vi "Regulator.vi"(8 "Odczyt odom":bool, 9 "Parametry regulatora":cluster{"kp":dbl, "k alfa":dbl, "k beta":dbl}, 10 "Odległość do punktu":dbl format="%#_13g", 11 "Kąt tryg. zad":dbl) -> (2 "w - prędkość kątowa":dbl, 3 "V - prędkość postępowa":dbl)   [LabVIEW 2015, in "Biblioteka moduł map v3.lvlib" / "Pomocnicze.lvlib"]
uses:
  Pomocnicze/Pomocnicze.lvlib
  Zmienne/szablon odometry_filtered_local.vi
  Zmienne/Zmienne.lvlib
  Matematyczne/Matematyczne.lvlib
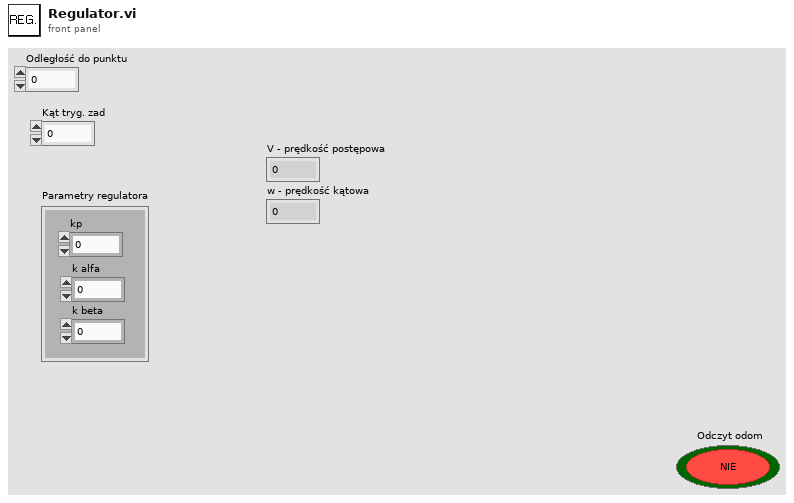
[diagram p1: front panel]
types:
  T1 = typedef "Biblioteka moduł map v3.lvlib/Zmienne.lvlib/szablon odometry_filtered_local.ctl" = cluster{"topic":string, "msg":cluster{"header":cluster{"seq":u32, "stamp":cluster{"secs":u32, "nsecs":i32}, "frame_id":string}, "child_frame_id":string, "pose":cluster{"pose":cluster{"position":cluster{"y":dbl, "z":dbl, "x":dbl}, "orientation":cluster{"y":dbl, "z":dbl, "x":dbl, "w":dbl}}, "covariance":dbl[]}, "twist":cluster{"twist":cluster{"linear":cluster{"y":dbl, "z":dbl, "x":dbl}, "angular":cluster{"y":dbl, "z":dbl, "x":dbl}}, "covariance":dbl[]}}, "op":string}
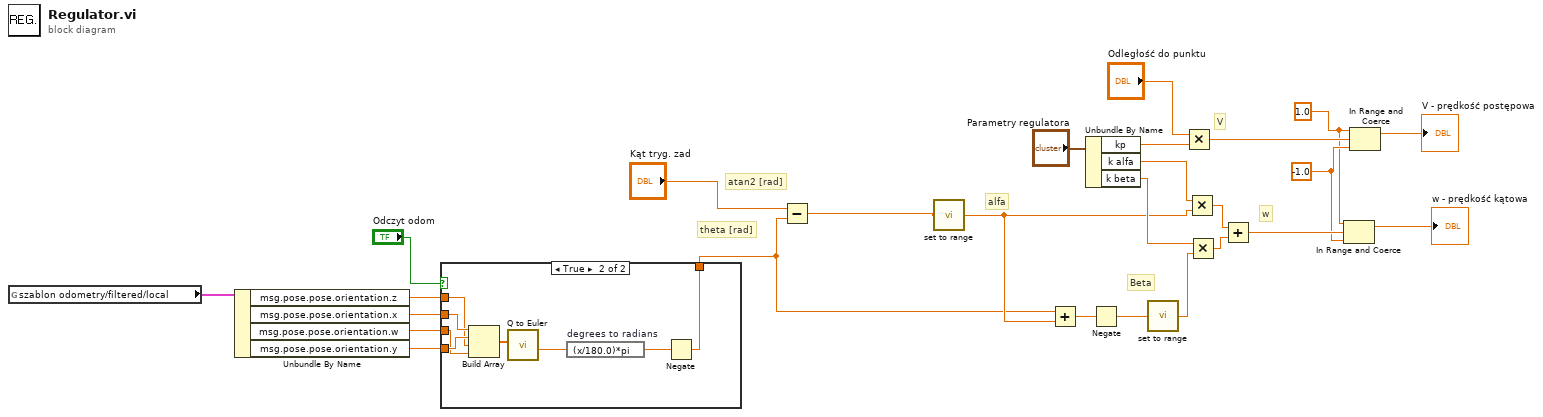
[diagram p0: block diagram]
diagram:
  w12 = 1.0 ("upper limit")
  w13 = -1.0 ("lower limit")
  # "w"
  # "V"
  # "Beta"
  # "atan2 [rad]"
  # "theta [rad]"
  # "alfa"
  n1 = global read "szablon odometry_filtered_local.vi" "szablon odometry/filtered/local"() -> (w17:T1)
  n2 = Unbundle By Name(w17) -> ("msg.pose.pose.orientation.z"=w4:dbl, "msg.pose.pose.orientation.x"=w6:dbl, "msg.pose.pose.orientation.w"=w3:dbl, "msg.pose.pose.orientation.y"=w5:dbl)
  n3 = case shown="True" "Odczyt odom" {
    tunnel: w6 -> [_ w35]
    tunnel: w5 -> [_ w34]
    tunnel: w4 -> [w27 w33]
    tunnel: w3 -> [_ w32]
    tunnel: [w27 w28] -> w2
    frame False {
    }
    frame True {
      n4 = Build Array(w35, w34, w33, w32) -> (w31:dbl[])
      n5 = call "Q to Euler.vi"("array"=w31) -> ("Yaw"=w30:dbl)  [unwired: 3 in, 3 out]
      n6 = expression code="(x/180.0)*pi" "degrees to radians"(w30) -> (w29:dbl)
      n7 = Negate(x=w29) -> (-x=w28:dbl)
    }
  }
  n8 = Subtract(x="Kąt tryg. zad", y=w2) -> (x-y=w10:dbl)
  n9 = call "set to range.vi"("kąt [rad]"=w10) -> ("kąt [rad] zredukowany"=w9:dbl)  [unwired: 4 in]
  n10 = Add(x=w2, y=w9) -> (x+y=w25:dbl)
  n11 = Unbundle By Name("Parametry regulatora") -> ("kp"=w22:dbl, "k alfa"=w19:dbl, "k beta"=w18:dbl)
  n12 = Negate(x=w25) -> (-x=w8:dbl)
  n13 = call "set to range.vi"("kąt [rad]"=w8) -> ("kąt [rad] zredukowany"=w7:dbl)  [unwired: 4 in]
  n14 = Multiply(x="Odległość do punktu", y=w22) -> (x*y=w16:dbl)
  n15 = Multiply(x=w19, y=w9) -> (x*y=w20:dbl)
  n16 = Multiply(x=w18, y=w7) -> (x*y=w21:dbl)
  n17 = Add(x=w20, y=w21) -> (x+y=w14:dbl)
  n18 = In Range and Coerce(upper limit=w12, x=w14, lower limit=w13) -> (coerced(x)=→"w - prędkość kątowa":dbl)  [unwired: 1 out]
  n19 = In Range and Coerce(upper limit=w12, x=w16, lower limit=w13) -> (coerced(x)=→"V - prędkość postępowa":dbl)  [unwired: 1 out]
